vi "Digitizer_Mode_TriggerRead.vi"(8 "error in":errorcluster, 11 "Channel Parameters In":T1) -> (0 "error out":errorcluster, 1 "Waveforms Out":T2(array[cluster]), 3 "dup Channel Parameters Out":T1)   [LabVIEW 2010]
uses:
  Typedef-Channel Parameters.ctl
  <instrlib>/niScope/Acquire/niScope Multi Read Cluster.vi
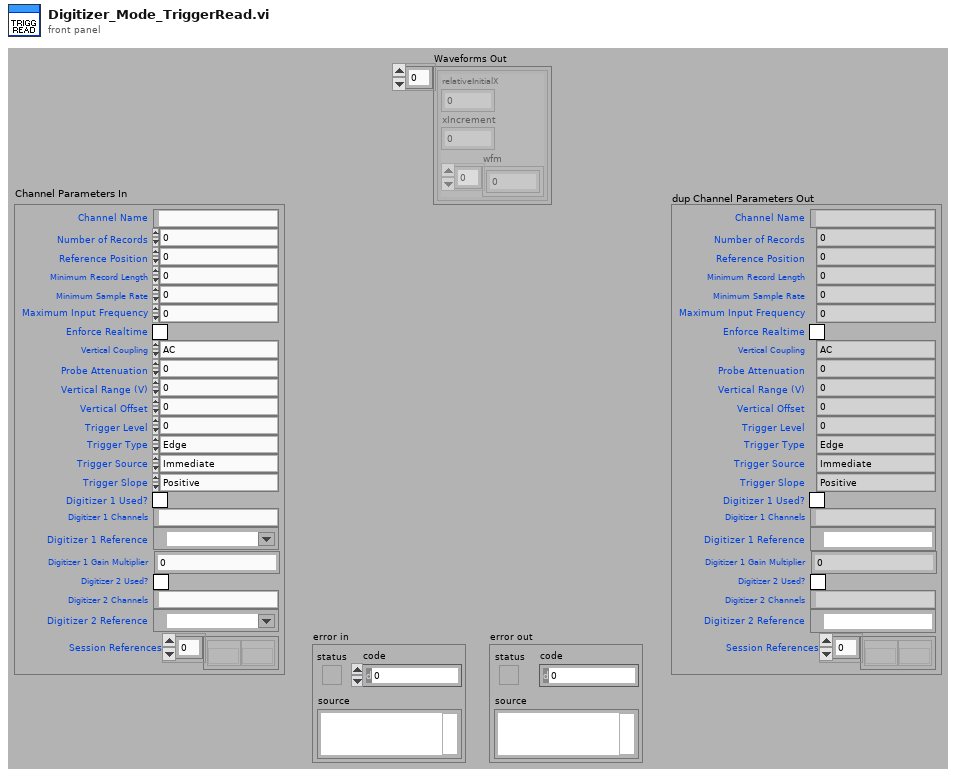
[diagram p1: front panel]
types:
  T1 = typedef "Typedef-Channel Parameters.ctl" = cluster{"Channel Name":string, "Number of Records":i32, "Reference Position":dbl, "Minimum Record Length":i32, "Minimum Sample Rate":dbl, "Maximum Input Frequency":dbl, "Enforce Realtime":bool, "Vertical Coupling":enum16{"AC", "DC", "Ground"}, "Probe Attenuation":dbl, "Vertical Range (V)":dbl, "Vertical Offset":dbl, "Trigger Level":dbl, "Trigger Type":enum16{"Edge", "Digital", "Immediate"}, "Trigger Source":enum16{"Immediate", "Channel 0", "Channel 1", "Channel 2", "Channel 3", "Channel 4", "Channel 5", "Channel 6", "Channel 7", "Extermal TRIG", "Software Trigger", "RTSI 0", "RTSI 1", "RTSI 2", "RTSI 3", "RTSI 4", "RTSI 5", "RTSI 6", "PF 0", "PF 1", "PF 2", "PXI Star Trigger"}, "Trigger Slope":enum16{"Positive", "Negative"}, "Digitizer 1 Used?":bool, "Digitizer 1 Channels":string, "Digitizer 1 Reference":refnum<k15>, "Digitizer 1 Gain Multiplier":dbl, "Digitizer 2 Used?":bool, "Digitizer 2 Channels":string, "Digitizer 2 Reference":refnum<k15>, "Session References":refnum<k20>[]}
  T2 = cluster{"relativeInitialX":dbl, "xIncrement":dbl, "wfm":dbl[]}[]
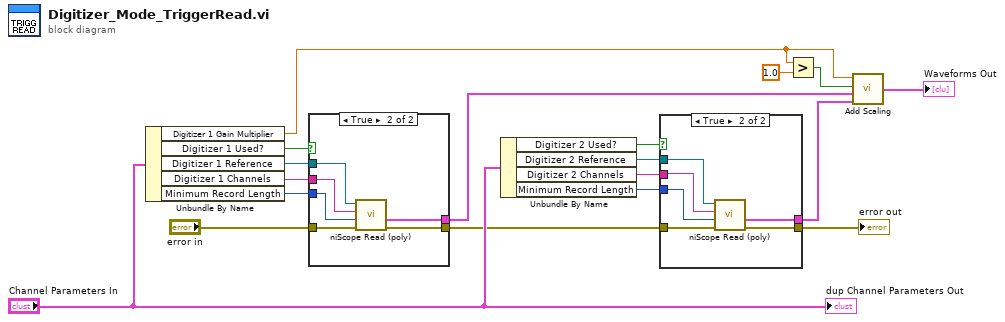
[diagram p0: block diagram]
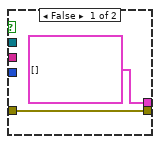
[diagram p2: hidden frame]
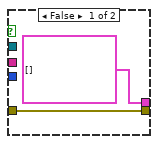
[diagram p3: hidden frame]
diagram:
  n1 = Unbundle By Name("Channel Parameters In") -> ("Digitizer 1 Gain Multiplier"=w17:dbl, "Digitizer 1 Used?"=w6:bool, "Digitizer 1 Reference"=w7:refnum<k15>, "Digitizer 1 Channels"=w8:string, "Minimum Record Length"=w9:i32)
  n2 = case shown="True" w6 {
    tunnel: w8 -> [_ w25]
    tunnel: "error in" -> [w20 w26]
    tunnel: w7 -> [_ w21]
    tunnel: [w20 w22] -> w4
    tunnel: [T2 [] ("waveform") w24] -> w3
    tunnel: w9 -> [_ w23]
    frame False {
    }
    frame True {
      n3 = call-poly <instrlib>:"niScope Read (poly).vi"("error in"=w26, "numSamples"=w23, "channels"=w25, "instrument handle"=w21) -> ("error out"=w22:errorcluster, "waveform"=w24:T2)  [unwired: 4 in, 2 out]
    }
  }
  n4 = Unbundle By Name("Channel Parameters In") -> ("Digitizer 2 Used?"=w11:bool, "Digitizer 2 Reference"=w12:refnum<k15>, "Digitizer 2 Channels"=w13:string, "Minimum Record Length"=w14:i32)
  n5 = case shown="True" w11 {
    tunnel: w13 -> [_ w30]
    tunnel: w4 -> [w28 w34]
    tunnel: w12 -> [_ w29]
    tunnel: w14 -> [_ w33]
    tunnel: [w28 w31] -> w5
    tunnel: [T2 [] ("waveform") w32] -> w1
    frame False {
    }
    frame True {
      n6 = call-poly <instrlib>:"niScope Read (poly).vi"("error in"=w34, "numSamples"=w33, "channels"=w30, "instrument handle"=w29) -> ("error out"=w31:errorcluster, "waveform"=w32:T2)  [unwired: 4 in, 2 out]
    }
  }
  "error out" <- w5
  n7 = Greater?(x=w17, y=1.0) -> (0:w18:bool)
  n8 = call "Add Scaling.vi"("Digitizer 2 Waveforms"=w1, "Digitizer 1 Waveforms"=w3, "Add Tegam Scaling?"=w18, "Digitizer 1 Gain Multiplier"=w17) -> ("Waveforms Out"=→"Waveforms Out":T2)
  "dup Channel Parameters Out" <- "Channel Parameters In"
